vi "Arduino LED test.vi"() -> ()   [LabVIEW 2025]
uses:
  8df395ab-0a8f-410c-933f-4c6911685367.vi
  <vilib>/Instr/_visa.llb/VISA Configure Serial Port (Instr).vi
panel:
  out "Response":string
  in  "stop":bool
  in  "OFF Button":bool
  in  "ON Button":bool
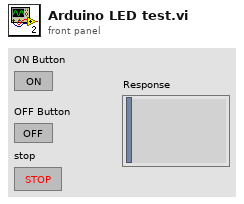
[diagram p1: front panel]
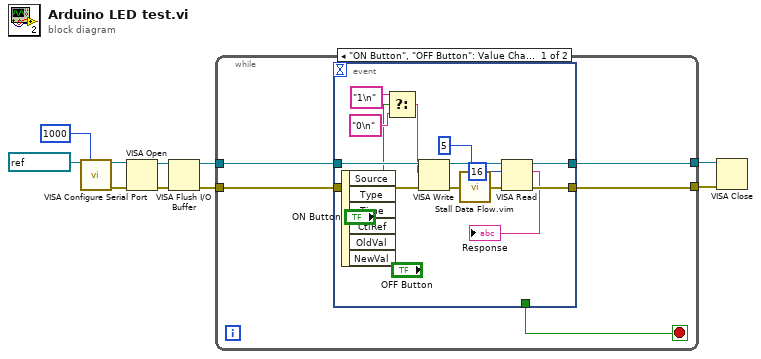
[diagram p0: block diagram]
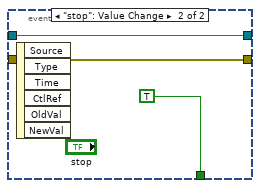
[diagram p2: hidden frame]
diagram:
  n1 = call-poly "VISA Configure Serial Port"("VISA resource name"=refnum<visa-resource-name> "COM3", "timeout (10sec)"=u32 1000) -> ("VISA resource name out"=w9:refnum<visa-resource-name>, "error out"=w10:errorcluster)  [unwired: 12 in]
  n2 = VISA Open(error in (no error)=w10, VISA resource name=w9) -> (VISA resource name=w2:refnum<visa-resource-name>, error out=w8:errorcluster)  [unwired: 3 in]
  n3 = VISA Flush I/O Buffer(VISA resource name=w2, error in (no error)=w8) -> (VISA resource name out=w1:refnum<visa-resource-name>, error out=w3:errorcluster)  [unwired: 1 in]
  n4 = while {
    tunnel: w3 -> [w14]
    tunnel: w1 -> [w15]
    tunnel: [w12] -> w7
    tunnel: [w13] -> w6
    stop <- w11 stop-if-true
    n5 = event shown="[0] \"ON Button\", \"OFF Button\": Value Change" {
      selector: _ -> [_ _]
      dyn-events: _ -> [_ _]
      timeout: _ -> [_ _]
      tunnel: w15 -> [w29 w32]
      tunnel: w14 -> [w28 w31]
      tunnel: [w24 w31] -> w13
      tunnel: [w23 w32] -> w12
      tunnel: [_ TRUE] -> w11
      event "ON Button", "OFF Button": Value Change {
        n6 = event-data() -> ()  [unwired: 1 in, 6 out]
        n7 = Select(t="1\n", s="ON Button", f="0\n") -> (s? t:f=w19:string)
        n8 = VISA Write(VISA resource name=w29, write buffer=w19, error in (no error)=w28) -> (VISA resource name out=w25:refnum<visa-resource-name>, error out=w27:errorcluster)  [unwired: 1 out]
        n9 = call "Stall Data Flow.vim"("value in"=w27, "milliseconds to wait"=u32 5) -> ("value out"=w17:errorcluster)  [unwired: 1 out]
        n10 = VISA Read(VISA resource name=w25, byte count=u32 16, error in (no error)=w17) -> (VISA resource name out=w23:refnum<visa-resource-name>, read buffer=→"Response":string, error out=w24:errorcluster)  [unwired: 1 out]
      }
      event "stop": Value Change {
        n11 = event-data() -> ()  [unwired: 1 in, 6 out]
      }
    }
  }
  n12 = VISA Close(VISA resource name=w7, error in (no error)=w6) -> ()  [unwired: 1 out]
